vi "Validate Instr CFG.vi"(8 "Error In":errorcluster, 11 "<JSON>":string) -> (0 "Error Out":errorcluster, 2 "Is Valid?":bool)   [LabVIEW 2024, in "Configuration UI Actor.lvlib" / "Configuration UI Actor.lvclass"]
uses:
  Configuration UI Actor.lvclass
  HAL/Configurations/CFG JSON/CFG JSON.lvclass
  HAL/Configurations/CFG Base/CFG Base.lvclass/CFG Base.ctl
  cb9ced8a-8a45-4182-8293-c1a5c9e4d2b8.vi
  cb9ced8a-8a45-4182-8293-c1a5c9e4d2b8.vi/a4169a97-72fc-4003-a778-603cf20cafa0.vi
  <vilib>/JDP Science/JSONtext/Find Item.vi
  <vilib>/JDP Science/JSONtext/Next JSON Value.vi
  <vilib>/JDP Science/JSONtext/String Subset.vi
  <vilib>/JDP Science/JSONtext/Parsing/Advance past next JSON Value (inlined COPY).vi
  <vilib>/JDP Science/JSONtext/Parsing/Advance past whitespace.vi
  <vilib>/JDP Science/JSONtext/Parsing/Advance past String.vi
  <vilib>/JDP Science/JSONtext/Parsing/Advance past Number.vi
  <vilib>/JDP Science/JSONtext/Parsing/Advance past Line Ending.vi
  <vilib>/JDP Science/JSONtext/Parsing/Parse Full Path or Item Name.vi
  <vilib>/JDP Science/JSONtext/Parsing/Advance past Array.vi
  <vilib>/JDP Science/JSONtext/Parsing/Advance past Object.vi
  <vilib>/JDP Science/JSONtext/support/Error Cluster From Code.vi
  <vilib>/JDP Science/JSONtext/Offset/Find Item Locations by Path.vi
  <vilib>/JDP Science/JSONtext/JSON text to Variant.vi
  <vilib>/Utility/error.llb/Error Cluster From Error Code.vi
  <vilib>/JDP Science/JSONtext/LVClass Serializer/JSONtext LVClass Serializer.lvclass
  HAL/Configurations/CFG Base/CFG Base.lvclass
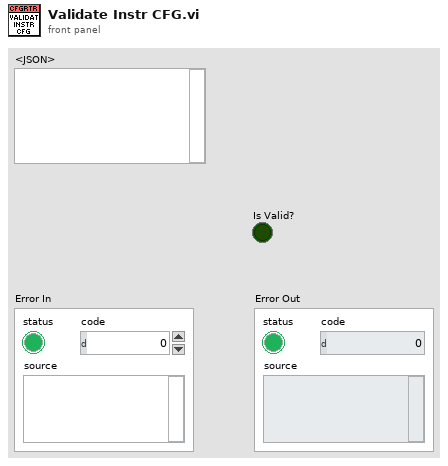
[diagram p1: front panel]
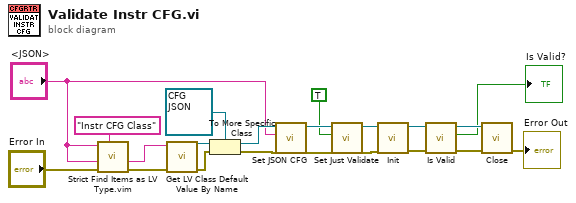
[diagram p0: block diagram]
diagram:
  n1 = call "Strict Find Items as LV Type.vim"("$Path or Item Name"="Instr CFG Class", "error in"="Error In", "Data Type and Default Value"="<JSON>", "<JSON>"="<JSON>") -> ("error out"=w19:errorcluster, "Data out"=w14:string)  [unwired: 5 in, 1 out]
  n2 = call <vilib>:"Get LV Class Default Value By Name.vi"("error in (no error)"=w19, "class name"=w14) -> ("error out"=w17:errorcluster, "object"=w16:refnum<class>)  [unwired: 8 in]
  n3 = To More Specific Class(target class=refnum<class "CFG JSON.lvclass"> refnum ("HAL.lvlib:CFG JSON.lvclass"), reference=w16, error in=w17) -> (specific class reference=w13:refnum<class "CFG JSON.lvclass">, error out=w2:errorcluster)
  n4 = call "Set JSON CFG.vi"("<JSON> CFG"="<JSON>", "CFG JSON in"=w13) -> ("CFG JSON out"=w6:refnum<class "CFG JSON.lvclass">)  [unwired: 9 in]
  n5 = call "Set Just Validate.vi"("Just Validate"=TRUE, "CFG Base in"=w6) -> ("CFG Base out"=w4:refnum<class "CFG JSON.lvclass">)  [unwired: 9 in]
  n6 = call-dynamic "Init.vi"("error in"=w2, "CFG Base in"=w4) -> ("error out"=w7:errorcluster, "CFG Base out"=w5:refnum<class "CFG JSON.lvclass">)  [unwired: 8 in]
  n7 = call-dynamic "Is Valid.vi"("error in"=w7, "CFG Base in"=w5) -> ("error out"=w10:errorcluster, "Valid"=→"Is Valid?":bool, "CFG Base out"=w8:refnum<class "CFG JSON.lvclass">)  [unwired: 7 in]
  n8 = call-dynamic "Close.vi"("error in"=w10, "CFG Base in"=w8) -> ("error out"=→"Error Out":errorcluster)  [unwired: 8 in, 1 out]
